vi "SubsystemWaitForCommand.vi"(7 "timeout/wait period (ms)":i32=10, 8 "error in (no error)":errorcluster, 11 "Queue in":refnum<queue>) -> (2 "timed out?":bool, 3 "DriveSubsystemCommand":T1)   [LabVIEW 2017]
uses:
  DriveCommand.ctl
  RunMode.ctl
  RobotSubsystem.lvclass
  SubsystemData/DriveData/DriveData.lvclass
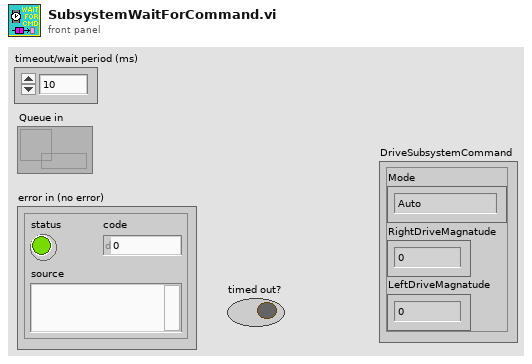
[diagram p1: front panel]
types:
  T1 = typedef "DriveData.lvclass/DriveCommand.ctl" = cluster{"Mode":T2, "RightDriveMagnatude":dbl, "LeftDriveMagnatude":dbl}
  T2 = typedef "RobotSubsystem.lvclass/RunMode.ctl" = enum16{"Auto", "Teleop", "Disabled"}
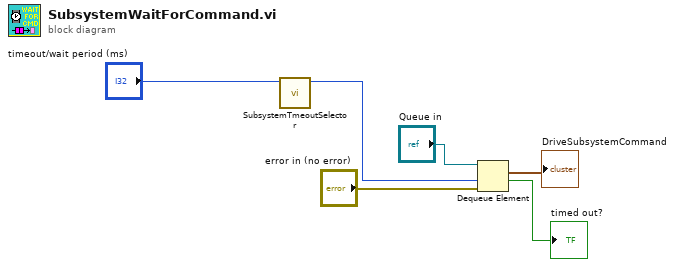
[diagram p0: block diagram]
diagram:
  n1 = call "SubsystemTmeoutSelector.vi"("timeout/wait period (ms)"="timeout/wait period (ms)") -> ("timeout to use"=w6:i32)  [unwired: 10 in]
  n2 = Dequeue Element(queue="Queue in", timeout in ms (-1)=w6, error in (no error)="error in (no error)") -> (element=→"DriveSubsystemCommand":T1, timed out?=→"timed out?":bool)  [unwired: 2 out]
